vi "AddNewMinMaxEntry.vi"(0 "Add New Entry?":bool, 5 "error in (no error)":errorcluster) -> (19 "error out":errorcluster)   [LabVIEW 2019, in "IndoorData.lvclass"]
uses:
  IndoorData.lvclass
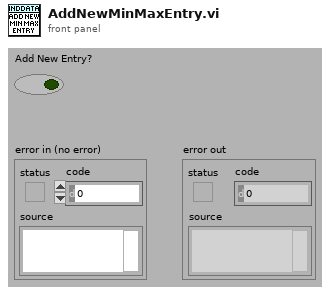
[diagram p1: front panel]
types:
  T1 = enum16{"open", "replace", "create", "open or create", "replace or create", "replace or create with confirmation"}
  T2 = typedef "IndoorData.lvclass/BufferedReadings.ctl" = cluster{"Time":dbl[], "Temp":dbl[], "RH":dbl[]}
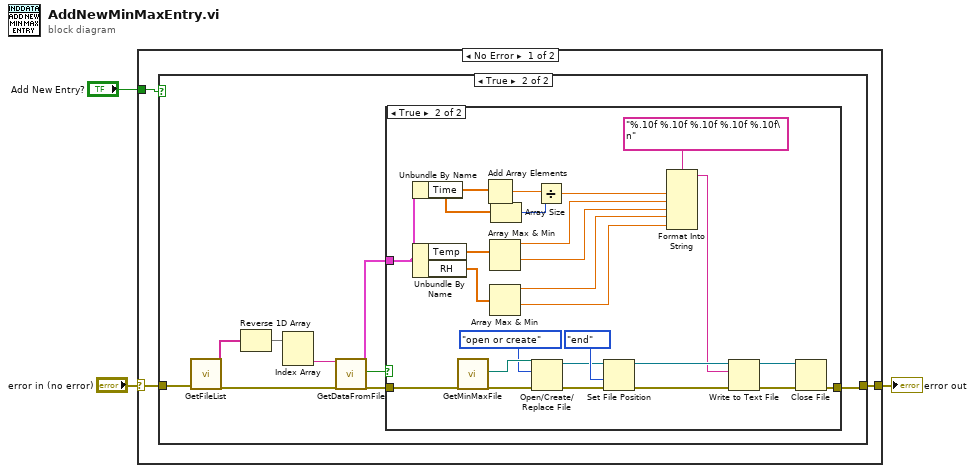
[diagram p0: block diagram]
diagram:
  n1 = case shown="No Error" "error in (no error)" {
    selector: "error in (no error)" -> [w6 w43]
    tunnel: [w4 w43] -> w2
    tunnel: "Add New Entry?" -> [w5 _]
    frame No Error {
      n2 = case shown="True" w5 {
        tunnel: w6 -> [w7 w16]
        tunnel: [w7 w9] -> w4
        frame False {
        }
        frame True {
          n3 = call "GetFileList.vi"("error in (no error)"=w16) -> ("filenames"=w15:string[], "error out"=w13:errorcluster)  [unwired: 17 in]
          n4 = Reverse 1D Array(array=w15) -> (reversed array=w14:string[])
          n5 = Index Array(array=w14) -> (element #2=w12:string)  [unwired: 2 in, 1 out]
          n6 = call "GetDataFromFile.vi"("FileName"=w12, "error in (no error)"=w13) -> ("FileData"=w11:T2, "file or folder exists?"=w8:bool, "error out"=w10:errorcluster)  [unwired: 15 in]
          n7 = case shown="True" w8 {
            tunnel: w11 -> [_ w31]
            tunnel: w10 -> [w17 w30]
            tunnel: [w17 w18] -> w9
            frame False {
            }
            frame True {
              n8 = Unbundle By Name(w31) -> ("Time"=w40:dbl[])
              n9 = Unbundle By Name(w31) -> ("Temp"=w41:dbl[], "RH"=w42:dbl[])
              n10 = call "GetMinMaxFile.vi"("error in (no error)"=w30) -> ("MinMaxFile"=w26:path, "error out"=w27:errorcluster)  [unwired: 17 in]
              n11 = Add Array Elements(numeric array=w40) -> (sum=w39:dbl)
              n12 = Array Max & Min(array=w41) -> (max value=w35:dbl, min value=w34:dbl)  [unwired: 2 out]
              n13 = Array Max & Min(array=w42) -> (max value=w33:dbl, min value=w32:dbl)  [unwired: 2 out]
              n14 = Array Size(array=w40) -> (size(s)=w38:i32)
              n15 = Open/Create/Replace File(file path (use dialog)=w26, error in=w27, operation (0:open)=T1."open or create") -> (refnum out=w28:refnum<file>, error out=w24:errorcluster)  [unwired: 3 in, 1 out]
              n16 = Divide(x=w39, y=w38) -> (x/y=w36:dbl)
              n17 = Set File Position(refnum=w28, from (0:start)=enum16{"start", "end", "current"}."end", error in=w24) -> (refnum out=w22:refnum<file>, error out=w23:errorcluster)  [unwired: 1 in]
              n18 = Format Into String(format string="%.10f %.10f %.10f %.10f %.10f\n", w36, w35, w34, w33, w32) -> (resulting string=w21:string)  [unwired: 2 in, 1 out]
              n19 = Write to Text File(file (use dialog)=w22, text=w21, error in=w23) -> (refnum out=w19:refnum<file>, error out=w20:errorcluster)  [unwired: 1 in, 1 out]
              n20 = Close File(refnum=w19, error in=w20) -> (error out=w18:errorcluster)  [unwired: 1 out]
            }
          }
        }
      }
    }
    frame Error {
    }
  }
  "error out" <- w2
